vi "Set IInstrument.vi"(8 "error in":errorcluster, 10 "IInstrument":refnum<class "IInstrument.lvclass">, 11 "NEO480 in":refnum<class "Virtual NEO480.lvclass">) -> (0 "error out":errorcluster, 3 "NEO480 out":refnum<class "Virtual NEO480.lvclass">)   [LabVIEW 2024, in "Virtual NEO480.lvclass"]
uses:
  Virtual NEO480.lvclass
  Source/Interfaces/IInstrument/IInstrument.lvclass
  Source/DBC Communicator/DBC Communicator.lvclass
  Virtual NEO480.lvclass/Virtual NEO480.ctl
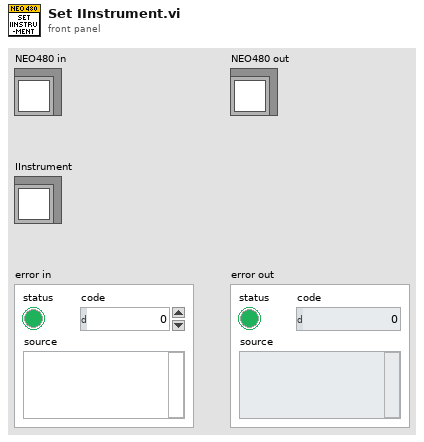
[diagram p1: front panel]
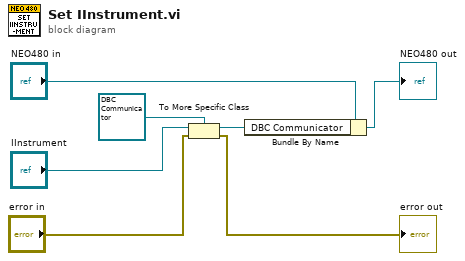
[diagram p0: block diagram]
diagram:
  n1 = To More Specific Class(target class=refnum<class "DBC Communicator.lvclass"> refnum ("DBC Communicator"), reference="IInstrument", error in="error in") -> (specific class reference=w5:refnum<class "DBC Communicator.lvclass">, error out=→"error out":errorcluster)
  n2 = Bundle By Name(cluster="NEO480 in", "DBC Communicator"=w5) -> (→"NEO480 out":refnum<class "Virtual NEO480.lvclass">)
